vi "Returning Values By Reference Integer.vi"(9 "sum":i32, 10 "y":i32, 11 "x":i32) -> (1 "sum out":i32)   [LabVIEW 2018, in "ParsingDataSampleDLL.lvlib"]
doc: "__declspec(dllexport) void ReturningValuesByReference_Integer (int x, int y, int *sum);"
uses:
  ParsingDataSampleDLL.lvlib
  ni_reference_vs/Debug/ParsingDataSampleDLL.dll
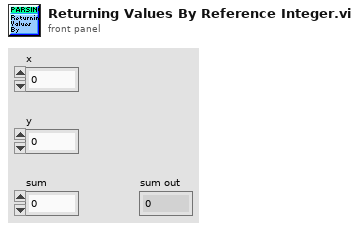
[diagram p1: front panel]
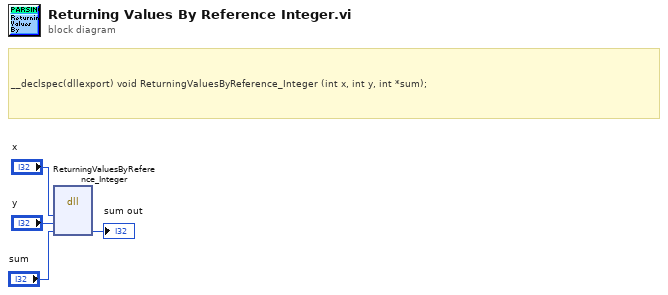
[diagram p0: block diagram]
diagram:
  # "__declspec(dllexport) void ReturningValuesByReference_Integer (int x, int y, int *sum);"
  n1 = dll-call lib="C:/Users/celit/Documents/GitHub/Labview_Python_DLL_Call/ni_reference_vs/Debug/ParsingDataSampleDLL.*" fn="ReturningValuesByReference_Integer"("x"="x", "y"="y", "sum"="sum") -> ("sum"=→"sum out":i32)  [unwired: 6 in, 2 out]
